vi "_stream Send Read.vi"(8 "error in":errorcluster, 10 "Response Data in":T1, 11 "Call ID in":T2) -> (0 "error out":errorcluster, 1 "Success":bool, 2 "Response Data out":T1, 3 "Call ID":T2)   [LabVIEW 2021, in "streamtest_client.lvlib"]
uses:
  streamtest_client.lvlib
  eef86c8b-2527-4d80-98ef-7d1dd29a9216.vi
  <vilib>/gRPC/LabVIEW gRPC Library/Shared/grpcId.ctl
  <vilib>/gRPC/LabVIEW gRPC Library/grpc-lvsupport-release.lvlib
  RPC Messages/streamtest_StreamData.ctl
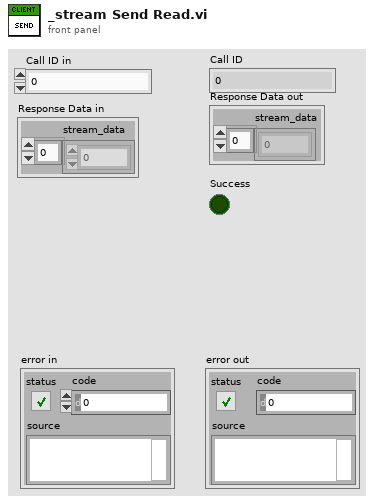
[diagram p1: front panel]
types:
  T1 = typedef "streamtest_client.lvlib/streamtest_StreamData.ctl" = cluster{"stream_data":u8[]}
  T2 = typedef "grpc-lvsupport-release.lvlib/grpcId.ctl" = u64
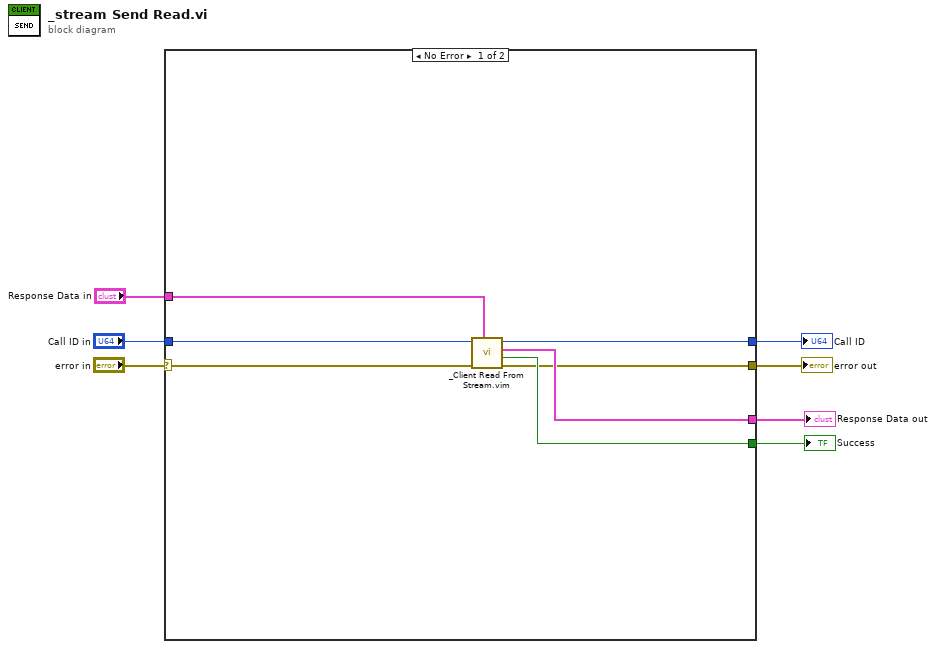
[diagram p0: block diagram]
diagram:
  n1 = case shown="No Error" "error in" {
    selector: "error in" -> [w12 w15]
    tunnel: [w8 w15] -> w6
    tunnel: "Call ID in" -> [w13 w16]
    tunnel: [w11 w16] -> w4
    tunnel: [w10 _] -> w3
    tunnel: [w9 _] -> w2
    tunnel: "Response Data in" -> [w14 _]
    frame No Error {
      n2 = call "_Client Read From Stream.vim"("Response Type"=w14, "error in"=w12, "Call ID in"=w13) -> ("error out"=w8:errorcluster, "Success"=w9:bool, "Response Data"=w10:T1, "Call ID out"=w11:u64)  [unwired: 5 in]
    }
    frame Error {
    }
  }
  "error out" <- w6
  "Call ID" <- w4
  "Response Data out" <- w3
  "Success" <- w2
